vi "calc_triangle_min_max.vi"(0 "Array":dbl[][](array[numeric])) -> (1 "Array 3":dbl[](array[numeric]), 2 "Array 2":dbl[](array[numeric]))   [LabVIEW 2011]
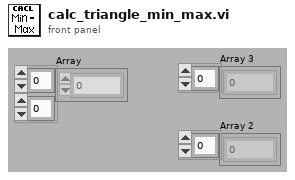
[diagram p1: front panel]
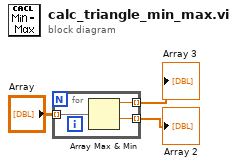
[diagram p0: block diagram]
diagram:
  n1 = for {
    tunnel: [w6] -> w1 mode=indexing
    tunnel: [w5] -> w2 mode=indexing
    tunnel: "Array" -> [w4] mode=indexing
    n2 = Array Max & Min(array=w4) -> (max value=w6:dbl, min value=w5:dbl)  [unwired: 2 out]
  }
  "Array 2" <- w2
  "Array 3" <- w1
